vi "Observe Data.vi"(6 "Time Stamp":timestamp, 8 "error in (no error)":errorcluster, 9 "Value":variant, 10 "Datum Name":string, 11 "SimpleChart in":refnum<class "SimpleChart.lvclass">) -> (0 "error out":errorcluster, 3 "SimpleChart out":refnum<class "SimpleChart.lvclass">)   [LabVIEW 2020, in "MVAExamples.lvlib" / "SimpleChart.lvclass"]
doc: "观察数据"
uses:
  SimpleChart.lvclass
  modules/mva-viewable/Source/IViewable/IViewable/IViewable.lvclass
panel:
  out "平均周期ms":dbl format="%#_6f"
  out "平均耗时ms":dbl format="%#_6f"
  out "周期ms":dbl format="%#_6f"
  out "发布到接收耗时ms":dbl format="%#_6f"
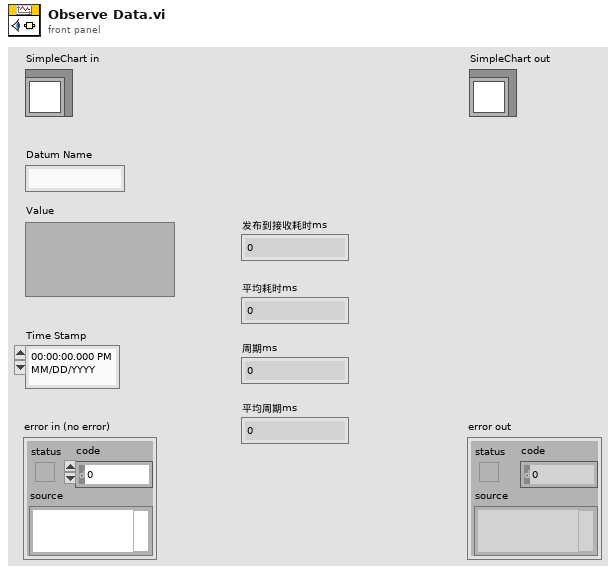
[diagram p1: front panel]
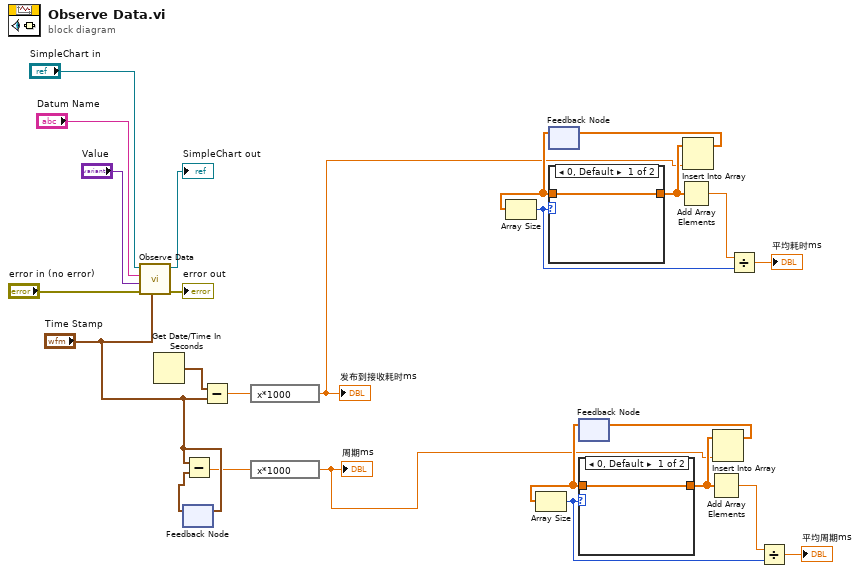
[diagram p0: block diagram]
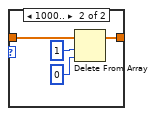
[diagram p2: hidden frame]
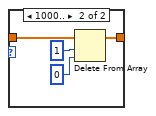
[diagram p3: hidden frame]
diagram:
  n1 = call-parent "Observe Data.vi"("Time Stamp"="Time Stamp", "error in (no error)"="error in (no error)", "Value"="Value", "Datum Name"="Datum Name", "IObserver in"="SimpleChart in") -> ("error out"=→"error out":errorcluster, "IObserver out"=→"SimpleChart out":refnum<class "SimpleChart.lvclass">)  [unwired: 5 in]
  n2 = Get Date/Time In Seconds() -> (seconds since 1Jan1904=w19:timestamp)
  n3 = feedback-in #1("Time Stamp") -> ()
  n4 = feedback #1() -> (w16:timestamp)  [unwired: 1 in]
  n5 = Subtract(x="Time Stamp", y=w16) -> (x-y=w15:dbl)
  n6 = Subtract(x=w19, y="Time Stamp") -> (x-y=w18:dbl)
  n7 = expression code="x*1000"(w18) -> (w9:dbl)
  "发布到接收耗时ms" <- w9
  n8 = expression code="x*1000"(w15) -> (w1:dbl)
  "周期ms" <- w1
  n9 = feedback #2() -> (w14:dbl[])  [unwired: 1 in]
  n10 = Array Size(array=w14) -> (size(s)=w10:i32)
  n11 = case shown="0, Default" w10 {
    tunnel: w14 -> [w26 w30]
    tunnel: [w26 w29] -> w12
    frame 0, Default {
    }
    frame 1000.. {
      n12 = Delete From Array(array=w30, length=1, index=0) -> (array with subset deleted=w29:dbl[])  [unwired: 1 out]
    }
  }
  n13 = feedback #3() -> (w2:dbl[])  [unwired: 1 in]
  n14 = Array Size(array=w2) -> (size(s)=w6:i32)
  n15 = case shown="0, Default" w6 {
    tunnel: w2 -> [w31 w35]
    tunnel: [w31 w34] -> w4
    frame 0, Default {
    }
    frame 1000.. {
      n16 = Delete From Array(array=w35, length=1, index=0) -> (array with subset deleted=w34:dbl[])  [unwired: 1 out]
    }
  }
  n17 = Add Array Elements(numeric array=w12) -> (sum=w11:dbl)
  n18 = Insert Into Array(array=w12, new element=w9) -> (w13:dbl[])  [unwired: 1 in]
  n19 = feedback-in #2(w13) -> ()
  n20 = Add Array Elements(numeric array=w4) -> (sum=w5:dbl)
  n21 = Insert Into Array(array=w4, new element=w1) -> (w3:dbl[])  [unwired: 1 in]
  n22 = feedback-in #3(w3) -> ()
  n23 = Divide(x=w11, y=w10) -> (x/y=→"平均耗时ms":dbl)
  n24 = Divide(x=w5, y=w6) -> (x/y=→"平均周期ms":dbl)
